vi "Write series.vi"(8 "error in (no error)":errorcluster, 10 "series":i32(ring) items=["AM", "H3U", "H5U"], 11 "InovanceSerialModbusRtu in":refnum<class "InovanceSerialModbusRtu.lvclass">) -> (0 "error out":errorcluster, 3 "InovanceSerialModbusRtu out":refnum<class "InovanceSerialModbusRtu.lvclass">)   [LabVIEW 2020, in "HslCommunication.lvlib" / "InovanceSerialModbusRtu.lvclass"]
uses:
  InovanceSerialModbusRtu.lvclass
  InovanceSerialModbusRtu.lvclass/InovanceSerialModbusRtu.ctl
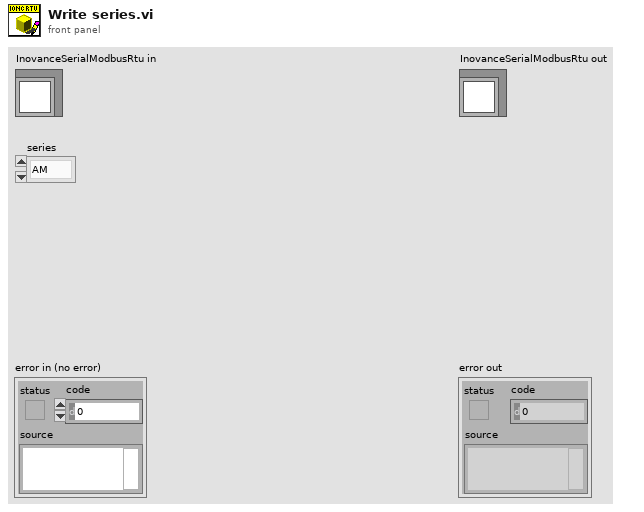
[diagram p1: front panel]
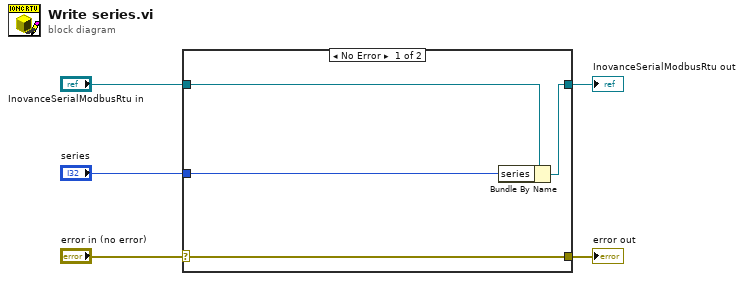
[diagram p0: block diagram]
diagram:
  n1 = case shown="No Error" "error in (no error)" {
    selector: "error in (no error)" -> [w9 w10]
    tunnel: [w9 w10] -> w4
    tunnel: [w7 w11] -> w2
    tunnel: "InovanceSerialModbusRtu in" -> [w8 w11]
    tunnel: "series" -> [w6 _]
    frame No Error {
      n2 = Bundle By Name(cluster=w8, "series"=w6) -> (w7:refnum<class "InovanceSerialModbusRtu.lvclass">)
    }
    frame Error {
    }
  }
  "error out" <- w4
  "InovanceSerialModbusRtu out" <- w2
